vi "Initialize FPGA.vi"(8 "error in (no error)":errorcluster, 11 "Simulation?":bool) -> (0 "error out":errorcluster, 3 "FPGA VI Reference":refnum<k20>)   [LabVIEW 2016]
uses:
  Typedefs/LV2G Operation.ctl
  Typedefs/IO Buffer Operation.ctl
  <vilib>/rvi/interface/RandomDataEmulation/nirviRandomDataOpen.vi
  <vilib>/rvi/interface/common/niFpgaCacheSessionInfoDynamic.vi
  <vilib>/FPGAPlugInAG/Dynamic/niLvFpga_Run_Dynamic.vi
  <vilib>/rvi/interface/nirviOpenFPGA/nirviOpenFPGA.xnode
  FPGA/FPGA_Main.vi
  <vilib>/rvi/interface/nirviMethod/nirviMethod.xnode
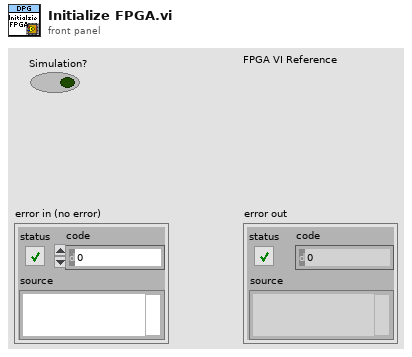
[diagram p1: front panel]
types:
  T1 = typedef "IO Buffer Operation.ctl" = enum16{"Initialize", "Write IO Data_Rd", "Read IO Data_Rd", "Write IO Data_Wr", "Read IO Data_Wr", "Write  IO Data_Dir", "Read  IO Data_Dir", "Write Host to Target FIFO", "Read Host to Target FIFO", "Write Target to Host FIFO", "Read Target to Host FIFO", "Write Monitor Enable?", "Read Monitor Enable?", "Close"}
  T2 = typedef "LV2G Operation.ctl" = enum16{"Initialize", "Set", "Get", "Close"}
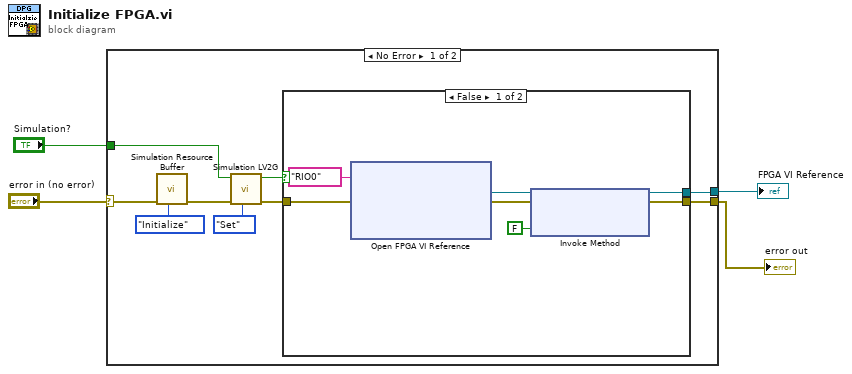
[diagram p0: block diagram]
diagram:
  n1 = case shown="No Error" "error in (no error)" {
    selector: "error in (no error)" -> [w7 w22]
    tunnel: [w8 w22] -> w3
    tunnel: [w13 _] -> w2
    tunnel: "Simulation?" -> [w9 _]
    frame No Error {
      n2 = call "Simulation Resource Buffer.vi"("IO Buffer Operation"=IO_Buffer_Operation."Initialize", "error in (no error)"=w7) -> ("error out"=w6:errorcluster)  [unwired: 7 in, 2 out]
      n3 = call "Simulation LV2G.vi"("Operation (Get)"=LV2G_Operation."Set", "error in (no error)"=w6, "Simulation?"=w9) -> ("error out"=w12:errorcluster, "Simulation? out"=w10:bool)  [unwired: 7 in]
      n4 = case shown="False" w10 {
        tunnel: w12 -> [w20 w21]
        tunnel: [w18 w21] -> w8
        tunnel: [w17 _] -> w13
        frame False {
          n5 = xnode "Open FPGA VI Reference"("error in"=w20, "resource name"=tag "RIO0") -> ("FPGA VI Reference Out"=w15:refnum<k20>, "error out"=w16:errorcluster)
          n6 = xnode "Invoke Method"("FPGA VI Reference In"=w15, "error in"=w16, "Wait Until Done (F)"=FALSE) -> ("FPGA VI Reference Out"=w17:refnum<k20>, "error out"=w18:errorcluster)
        }
        frame True {
        }
      }
    }
    frame Error {
    }
  }
  "error out" <- w3
  "FPGA VI Reference" <- w2
